vi "Interfazdelacortina.vi"() -> ()   [LabVIEW 2025]
uses:
  <vilib>/Instr/_visa.llb/VISA Configure Serial Port (Instr).vi
panel:
  in  "PARO DE \nEMERGENCIA":bool
  out "Señal Arduino":string
  out "Dirección de Anvance":string
  in  "ARRIBA":bool
  in  "ABAJO":bool
  out "Cortina":dbl(slide) scale=0.0..10.0
  out "Modo Seleccionado":string
  in  "MODO":bool
  in  "VISA resource name":refnum<visa-resource-name>
  in  "stop":bool
  # "Automatico"
  # "Manual"
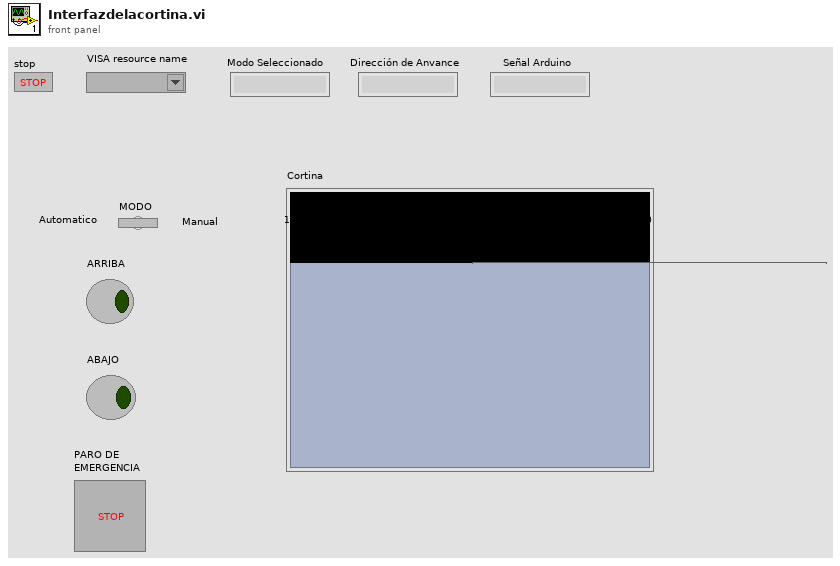
[diagram p1: front panel]
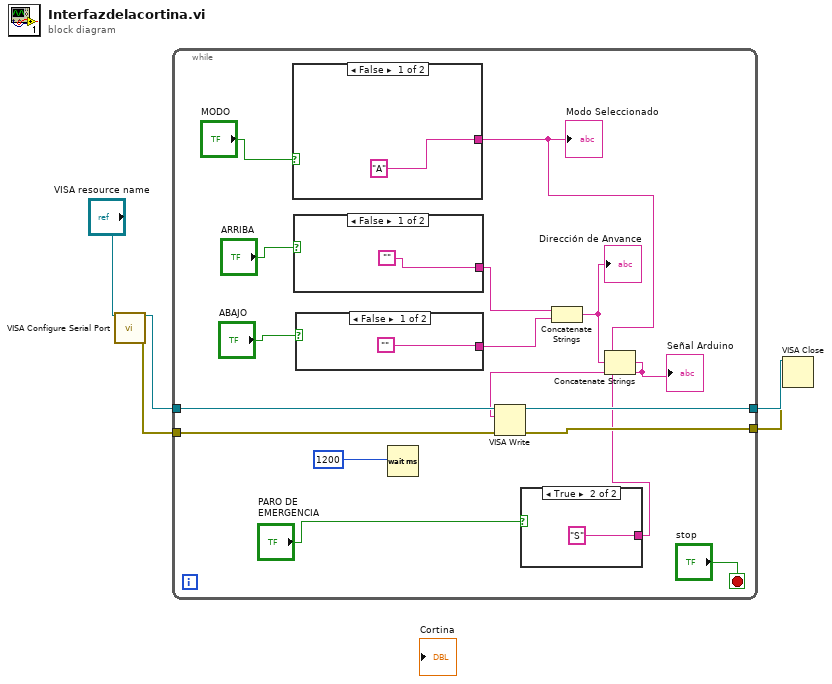
[diagram p0: block diagram]
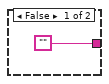
[diagram p2: hidden frame]
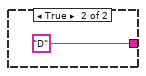
[diagram p3: hidden frame]
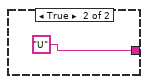
[diagram p4: hidden frame]
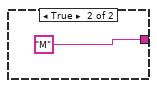
[diagram p5: hidden frame]
diagram:
  n1 = call-poly "VISA Configure Serial Port"("VISA resource name"="VISA resource name") -> ("VISA resource name out"=w4:refnum<visa-resource-name>, "error out"=w3:errorcluster)  [unwired: 13 in]
  n2 = while {
    tunnel: w4 -> [w21]
    tunnel: w3 -> [w20]
    tunnel: [w19] -> w2
    tunnel: [w18] -> w1
    stop <- "stop" stop-if-true
    n3 = case shown="False" "MODO" {
      tunnel: ["A" "M"] -> w11
      frame False {
      }
      frame True {
      }
    }
    "Modo Seleccionado" <- w11
    n4 = case shown="False" "ARRIBA" {
      tunnel: ["" "U"] -> w12
      frame False {
      }
      frame True {
      }
    }
    n5 = case shown="False" "ABAJO" {
      tunnel: ["" "D"] -> w13
      frame False {
      }
      frame True {
      }
    }
    n6 = Wait (ms)(milliseconds to wait=1200) -> ()  [unwired: 1 out]
    n7 = case shown="True" "PARO DE \nEMERGENCIA" {
      tunnel: ["" "S"] -> w7
      frame False {
      }
      frame True {
      }
    }
    n8 = Concatenate Strings(w12, w13) -> (w10:string)
    "Dirección de Anvance" <- w10
    n9 = Concatenate Strings(w11, w10, w7) -> (w9:string)
    "Señal Arduino" <- w9
    n10 = VISA Write(VISA resource name=w21, write buffer=w9, error in (no error)=w20) -> (VISA resource name out=w19:refnum<visa-resource-name>, error out=w18:errorcluster)  [unwired: 1 out]
  }
  n11 = VISA Close(VISA resource name=w2, error in (no error)=w1) -> ()  [unwired: 1 out]
